vi "NTC T2R_regi.vi"(8 "C=":dbl=1.537008174356433e-07, 9 "B=":dbl=0.0002616790491518455, 10 "A=":dbl=0.0012923134451485576, 11 "T [°C]":dbl) -> (3 "R [Ohm]":dbl)   [LabVIEW 2014]
panel:
  # "--->"
  # "A default értékek 2k-s\nNTC-re vonatkoznak."
  # "Steinhart-Hart egyenlet: \n1/T[K]=A+B*ln(R[Ohm])+C*(ln(R[Ohm))^3"
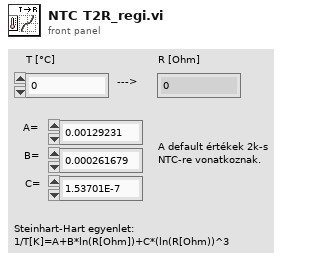
[diagram p1: front panel]
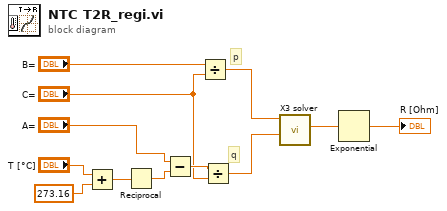
[diagram p0: block diagram]
diagram:
  # "q"
  # "p"
  n1 = Add(x="T [°C]", y=273.16) -> (x+y=w11:dbl)
  n2 = Reciprocal(x=w11) -> (1/x=w10:dbl)
  n3 = Subtract(x="A=", y=w10) -> (x-y=w8:dbl)
  n4 = Divide(x="B=", y="C=") -> (x/y=w4:dbl)
  n5 = Divide(x=w8, y="C=") -> (x/y=w3:dbl)
  n6 = call "X3 solver.vi"("q"=w3, "p"=w4) -> ("X"=w5:dbl)  [unwired: 9 in]
  n7 = Exponential(1:w5) -> (0:→"R [Ohm]":dbl)
